vi "14_1.vi"() -> ()   [LabVIEW 2018]
uses:
  <userlib>/_OpenG.lib/dictionary/dictionary.llb/Dictionary Update (by scalar value)__ogtk.vi
panel:
  out "sum":u64
  out "Array":u64[](array[numeric])
  out "items":cluster{"key":variant, "value":variant}[](array[cluster])
  out "Mask":string[](array[string])
  out "array":string[](array[string])
  in  "Input":string
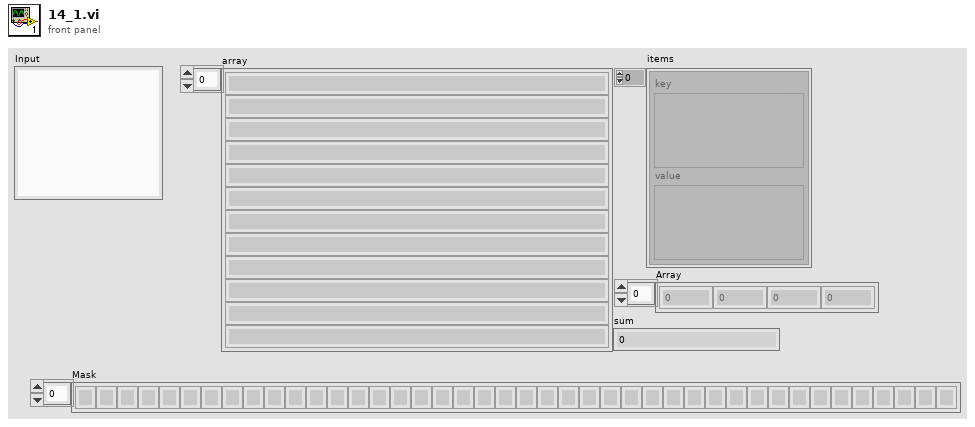
[diagram p1: front panel]
types:
  T1 = typedef "Dictionary Object RefNum__ogtk.ctl" = refnum<k1>
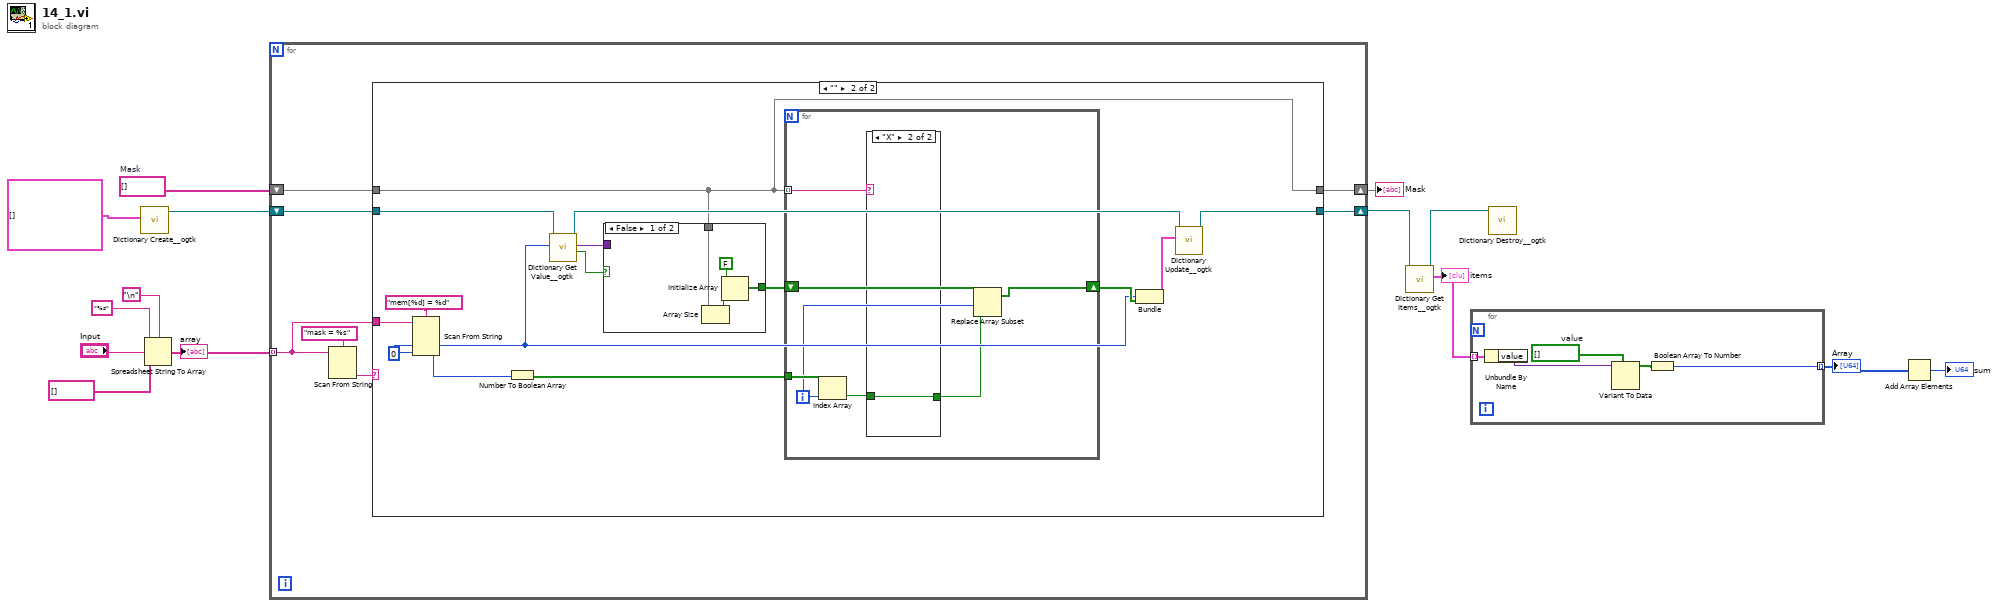
[diagram p0: block diagram]
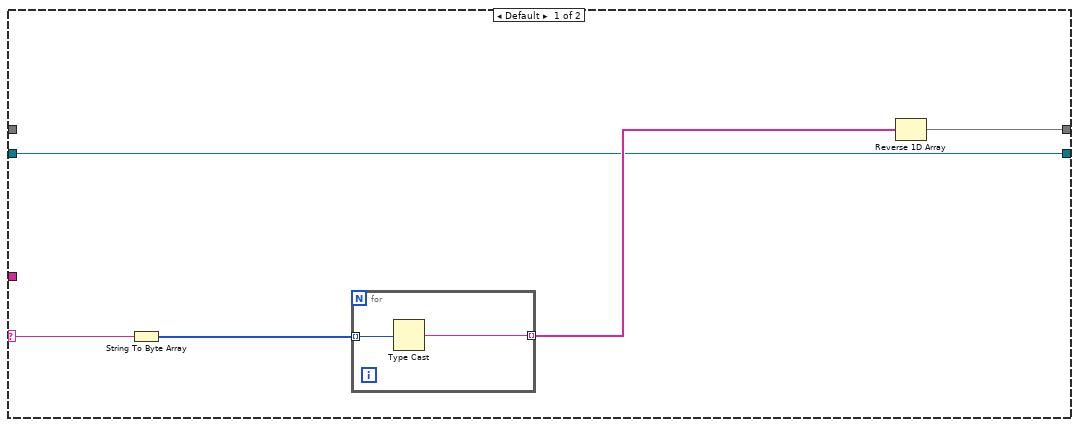
[diagram p2: hidden frame]
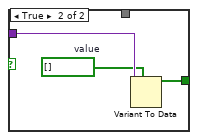
[diagram p3: hidden frame]
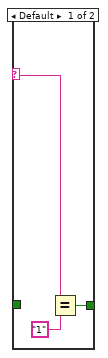
[diagram p4: hidden frame]
diagram:
  w9 = string[] []  # Mask
  n1 = call <userlib>:"Dictionary Create__ogtk.vi"("initial dictionary (empty)"=cluster{"key":u64, "value":bool[]}[] []) -> ("dictionary out"=w7:T1)  [unwired: 9 in, 1 out]
  n2 = Spreadsheet String To Array(delimiter (Tab)="\n", format string="%s", spreadsheet string="Input", array type (2D Dbl)=string[] []) -> (array=w10:string[])
  "array" <- w10
  n3 = for {
    tunnel: w10 -> [w15] mode=indexing
    shift-right: [w18] -> w8
    shift-left: w9 -> [w19]
    shift-right: [w16] -> w5
    shift-left: w7 -> [w17]
    n4 = Scan From String(format string="mask = %s", input string=w15) -> (output 1=w20:string)  [unwired: 3 in, 3 out]
    n5 = case shown="\"\"" w20 {
      selector: w20 -> [w26 _]
      tunnel: w19 -> [_ w32]
      tunnel: [w22 w32] -> w18
      tunnel: w17 -> [w23 w37]
      tunnel: [w23 w41] -> w16
      tunnel: w15 -> [_ w43]
      frame Default {
        n6 = String To Byte Array(string=w26) -> (unsigned byte array=w25:u8[])
        n7 = for {
          tunnel: w25 -> [w28] mode=indexing
          tunnel: [w27] -> w24 mode=indexing
          n8 = Type Cast(x=w28) -> (*(type *) &x=w27:string)  [unwired: 1 in]
        }
        n9 = Reverse 1D Array(array=w24) -> (reversed array=w22:string[])
      }
      frame "" {
        w29 = u64 0
        n10 = Scan From String(format string="mem[%d] = %d", input string=w43, default 1=w29, default 2=w29) -> (output 1=w38:u64, output 2=w30:u64)  [unwired: 2 in, 3 out]
        n11 = Number To Boolean Array(number=w30) -> (Boolean array=w31:bool[])
        n12 = call <userlib>:"Dictionary Get Value__ogtk.vi"("key"=w38, "dictionary"=w37) -> ("found?"=w33:bool, "value"=w36:variant, "dictionary out"=w34:T1)  [unwired: 6 in, 1 out]
        n13 = case shown="False" w33 {
          tunnel: w36 -> [_ w50]
          tunnel: w32 -> [w45 _]
          tunnel: [w47 w49] -> w35
          frame False {
            n14 = Array Size(array=w45) -> (size(s)=w46:i32)
            n15 = Initialize Array(FALSE, w46) -> (w47:bool[])
          }
          frame True {
            w48 = bool[] []  # value
            n16 = Variant To Data(type=w48, Variant=w50) -> (data=w49:bool[])  [unwired: 1 in, 1 out]
          }
        }
        n17 = for {
          tunnel: w32 -> [w57] mode=indexing
          tunnel: w31 -> [w55]
          shift-right: [w52] -> w40
          shift-left: w35 -> [w54]
          i -> [w51]
          n18 = Index Array(array=w55, index=w51) -> (element=w56:bool)
          n19 = case shown="\"X\"" w57 {
            selector: w57 -> [w60 _]
            tunnel: [w59 w61] -> w53
            tunnel: w56 -> [_ w61]
            frame Default {
              n20 = Equal?(x=w60, y="1") -> (x = y?=w59:bool)
            }
            frame "X" {
            }
          }
          n21 = Replace Array Subset(array=w54, new element=w53, index=w51) -> (w52:bool[])
        }
        n22 = Bundle(w38, "value"=w40) -> (w39:cluster{u64, "value":bool[]})  [unwired: 1 in]
        n23 = call-poly <userlib>:"Dictionary Update__ogtk.vi"("key-value"=w39, "dictionary"=w34) -> ("dictionary out"=w41:T1)  [unwired: 7 in, 2 out]
      }
    }
  }
  "Mask" <- w8
  n24 = call <userlib>:"Dictionary Get Items__ogtk.vi"("dictionary"=w5) -> ("items"=w3:cluster{"key":variant, "value":variant}[], "dictionary out"=w4:T1)  [unwired: 8 in, 1 out]
  "items" <- w3
  n25 = for {
    tunnel: w3 -> [w66] mode=indexing
    tunnel: [w62] -> w2 mode=indexing
    w65 = bool[] []  # value
    n26 = Unbundle By Name(w66) -> ("value"=w64:variant)
    n27 = Variant To Data(type=w65, Variant=w64) -> (data=w63:bool[])  [unwired: 1 in, 1 out]
    n28 = Boolean Array To Number(Boolean array=w63) -> (number=w62:u64)
  }
  "Array" <- w2
  n29 = call <userlib>:"Dictionary Destroy__ogtk.vi"("dictionary"=w4) -> ()  [unwired: 10 in, 1 out]
  n30 = Add Array Elements(numeric array=w2) -> (sum=→"sum":u64)
